vi "Errror on bit.vi"(8 "error in (no error)":errorcluster, 11 "ISO 14443 B UP in":refnum<class "ISO 14443 B UP.lvclass">) -> (0 "error out":errorcluster, 2 "Error on  byte":dbl, 3 "ISO 14443 B UP out":refnum<class "ISO 14443 B UP.lvclass">)   [LabVIEW 2019, in "ISO 14443 B UP.lvclass"]
uses:
  ISO 14443 B UP.lvclass
  ISO 14443 B UP.lvclass/ISO 14443 B UP.ctl
  <userlib>/_OpenG.lib/array/array.llb/Filter 1D Array with Scalar (Boolean)__ogtk.vi
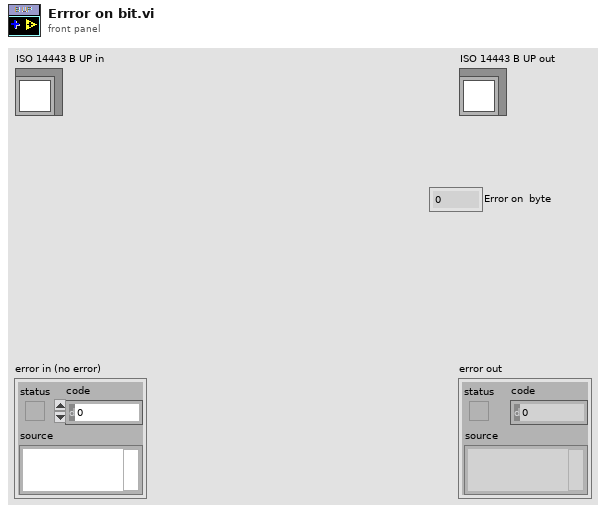
[diagram p1: front panel]
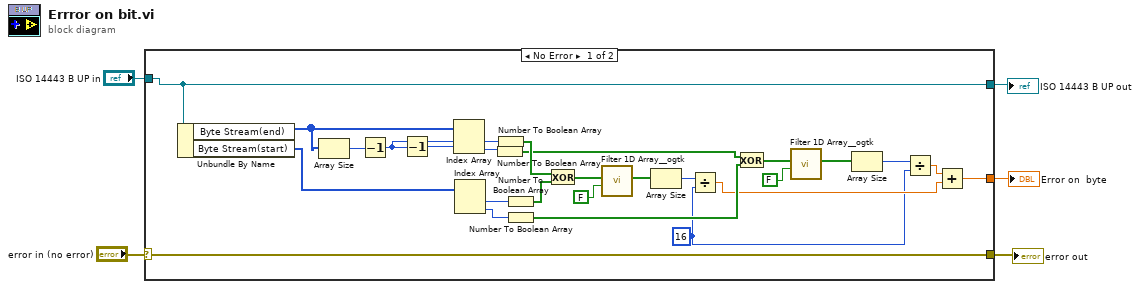
[diagram p0: block diagram]
diagram:
  n1 = case shown="No Error" "error in (no error)" {
    selector: "error in (no error)" -> [w32 w34]
    tunnel: "ISO 14443 B UP in" -> [w31 w33]
    tunnel: [w31 w33] -> w1
    tunnel: [w32 w34] -> w3
    tunnel: [w9 _] -> w2
    frame No Error {
      w6 = 16 ("y")
      n2 = Unbundle By Name(w31) -> ("Byte Stream(end)"=w21:u8[], "Byte Stream(start)"=w22:u8[])
      n3 = Array Size(array=w21) -> (size(s)=w20:i32)
      n4 = Decrement(x=w20) -> (x-1=w8:i32)
      n5 = Decrement(x=w8) -> (x-1=w7:i32)
      n6 = Index Array(array=w21, index #1=w8, index #2=w7) -> (element #1=w29:u8, element #2=w18:u8)
      n7 = Index Array(array=w22) -> (element #1=w30:u8, element #2=w19:u8)  [unwired: 2 in]
      n8 = Number To Boolean Array(number=w18) -> (Boolean array=w15:bool[])
      n9 = Number To Boolean Array(number=w29) -> (Boolean array=w28:bool[])
      n10 = Number To Boolean Array(number=w30) -> (Boolean array=w27:bool[])
      n11 = Number To Boolean Array(number=w19) -> (Boolean array=w14:bool[])
      n12 = Exclusive Or(1:w27, 2:w28) -> (0:w26:bool[])
      n13 = call-poly <userlib>:"Filter 1D Array__ogtk.vi"("items to filter"=FALSE, "array"=w26) -> ("filtered array"=w24:bool[])  [unwired: 4 in, 1 out]
      n14 = Array Size(array=w24) -> (size(s)=w23:i32)
      n15 = Divide(x=w23, y=w6) -> (x/y=w10:dbl)
      n16 = Exclusive Or(1:w14, 2:w15) -> (0:w16:bool[])
      n17 = call-poly <userlib>:"Filter 1D Array__ogtk.vi"("items to filter"=FALSE, "array"=w16) -> ("filtered array"=w12:bool[])  [unwired: 4 in, 1 out]
      n18 = Array Size(array=w12) -> (size(s)=w13:i32)
      n19 = Divide(x=w13, y=w6) -> (x/y=w11:dbl)
      n20 = Add(x=w11, y=w10) -> (x+y=w9:dbl)
    }
    frame Error {
    }
  }
  "error out" <- w3
  "ISO 14443 B UP out" <- w1
  "Error on  byte" <- w2
